vi "Scripting_ReplaceSubVI.vi"(8 "error in":errorcluster, 10 "NewVIToReplaceWith":path, 11 "CurrentSubVI":refnum<vi>) -> (0 "error out":errorcluster, 3 "ReplacedObject(SubVI)":refnum<vi>)   [LabVIEW 2016]
uses:
  <vilib>/Utility/miscctls.llb/LVPositionTypeDef.ctl
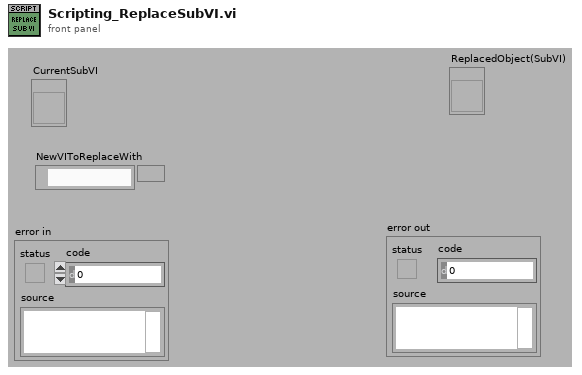
[diagram p1: front panel]
types:
  T1 = typedef "LVPositionTypeDef.ctl" = cluster{"Left":i32, "Top":i32}
  T2 = cluster{"ReplacedObject(SubVI)":refnum<vi>, "TerminalsOnCurrentSubVI":cluster{"Terminal":refnum<vi>, "Wire":refnum<vi>, "Position":T1, "IsSource":bool, "Data Type":variant, "WTerminals[]":refnum<vi>[]}[], "TerminalsOnNewSubVI":cluster{"Terminal":refnum<vi>, "Wire":refnum<vi>, "Position":T1, "IsSource":bool, "Data Type":variant, "WTerminals[]":refnum<vi>[]}[], "RepaireTerminals":cluster{"Org":cluster{"Terminal":refnum<vi>, "Wire":refnum<vi>, "Position":T1, "IsSource":bool, "Data Type":variant, "WTerminals[]":refnum<vi>[]}, "New":cluster{"Terminal":refnum<vi>, "Wire":refnum<vi>, "Position":T1, "IsSource":bool, "Data Type":variant, "WTerminals[]":refnum<vi>[]}}[]}
  T3 = cluster{"Terminal":refnum<vi>, "Wire":refnum<vi>, "Position":T1, "IsSource":bool, "Data Type":variant, "WTerminals[]":refnum<vi>[]}[]
  T4 = cluster{cluster{"Terminal":refnum<vi>, "Wire":refnum<vi>, "Position":T1, "IsSource":bool, "Data Type":variant, "WTerminals[]":refnum<vi>[]}, cluster{"Terminal":refnum<vi>, "Wire":refnum<vi>, "Position":T1, "IsSource":bool, "Data Type":variant, "WTerminals[]":refnum<vi>[]}}[]
  T5 = cluster{refnum<vi>, "Wire":refnum<vi>, "Position":T1, "IsSource":bool, "Data Type":variant, "Terms[]":refnum<vi>[]}
  T6 = cluster{"Terminal":refnum<vi>, "Wire":refnum<vi>, "Position":T1, "IsSource":bool, "Data Type":variant, "Terms[]":refnum<vi>[]}[]
  T7 = cluster{"Terminal":refnum<vi>, "Wire":refnum<vi>, "Position":T1, "IsSource":bool, "Data Type":variant, "WTerminals[]":refnum<vi>[]}
  T8 = cluster{cluster{"Terminal":refnum<vi>, "Wire":refnum<vi>, "Position":T1, "IsSource":bool, "Data Type":variant, "WTerminals[]":refnum<vi>[]}, cluster{"Terminal":refnum<vi>, "Wire":refnum<vi>, "Position":T1, "IsSource":bool, "Data Type":variant, "WTerminals[]":refnum<vi>[]}}
  T9 = cluster{"Org":cluster{"Terminal":refnum<vi>, "Wire":refnum<vi>, "Position":T1, "IsSource":bool, "Data Type":variant, "WTerminals[]":refnum<vi>[]}, "New":cluster{"Terminal":refnum<vi>, "Wire":refnum<vi>, "Position":T1, "IsSource":bool, "Data Type":variant, "WTerminals[]":refnum<vi>[]}}[]
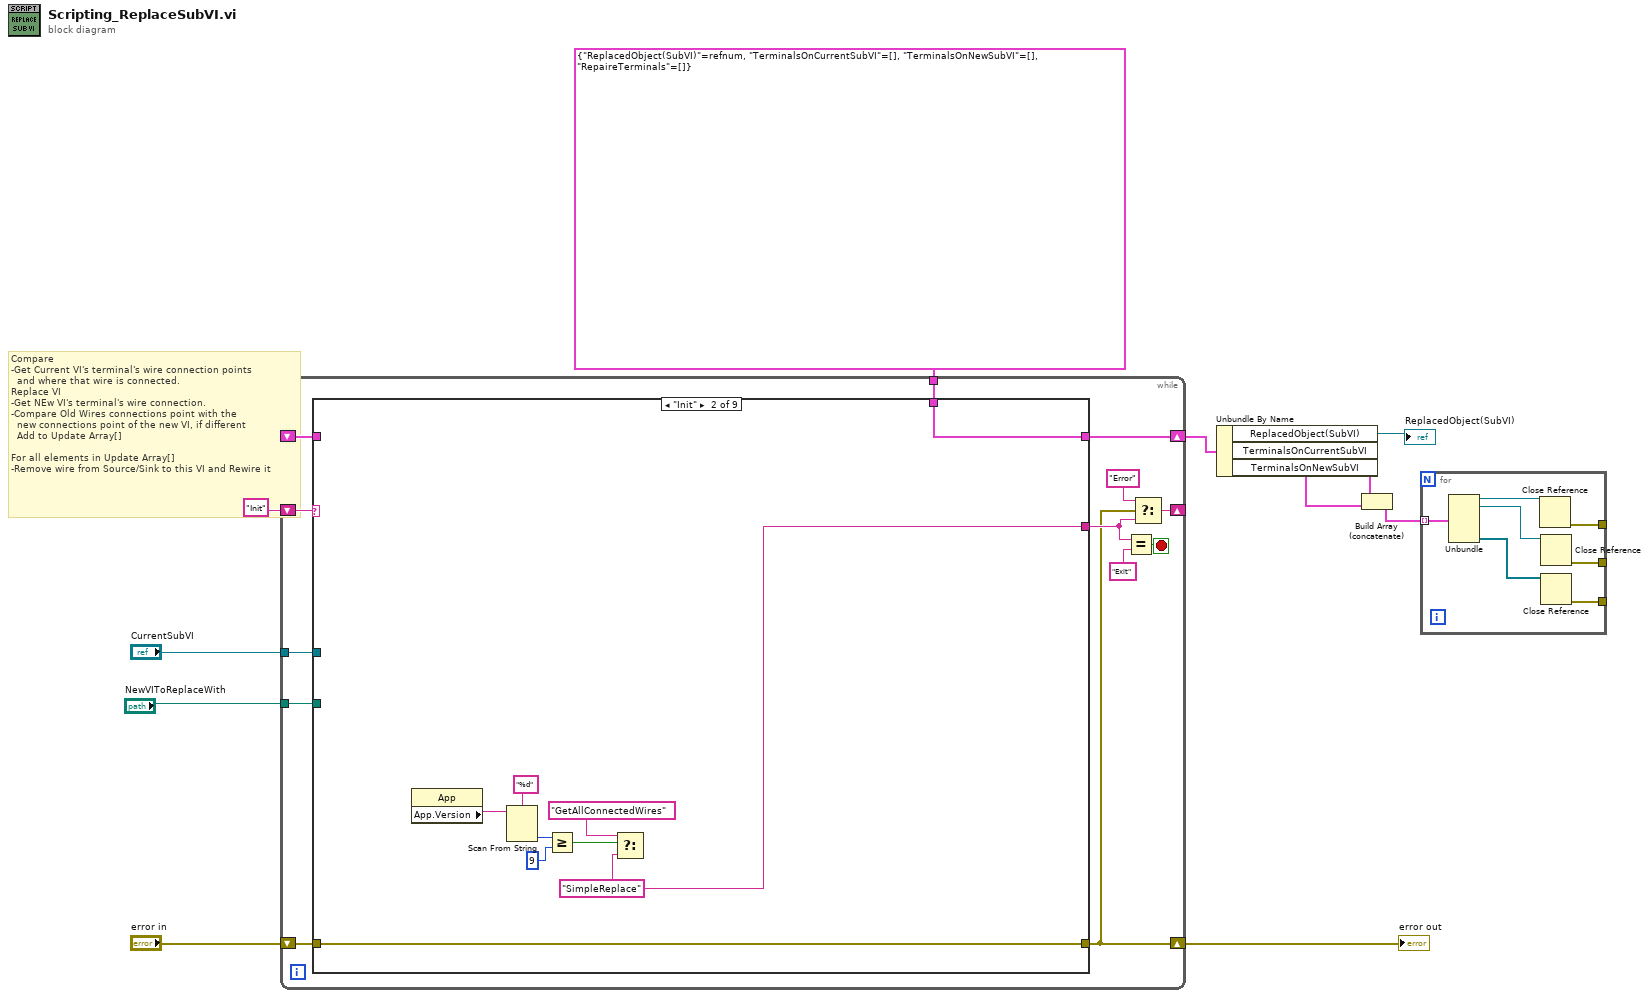
[diagram p0: block diagram]
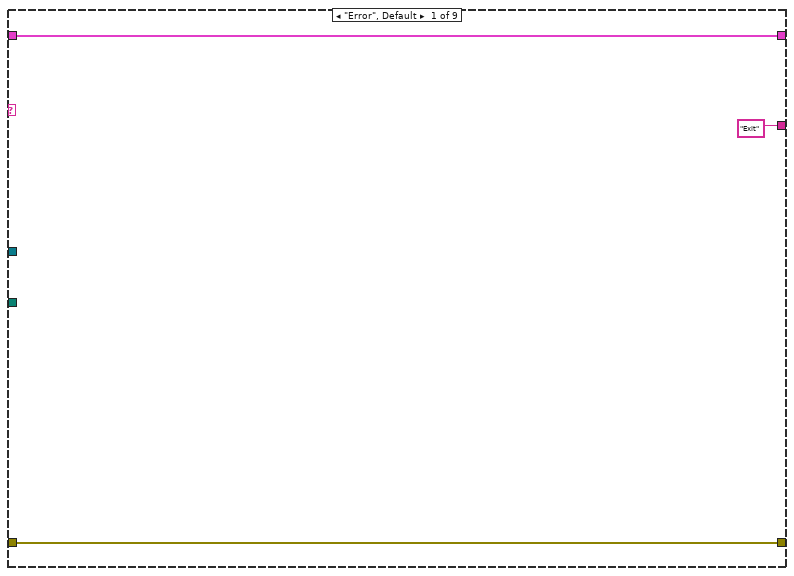
[diagram p2: hidden frame]
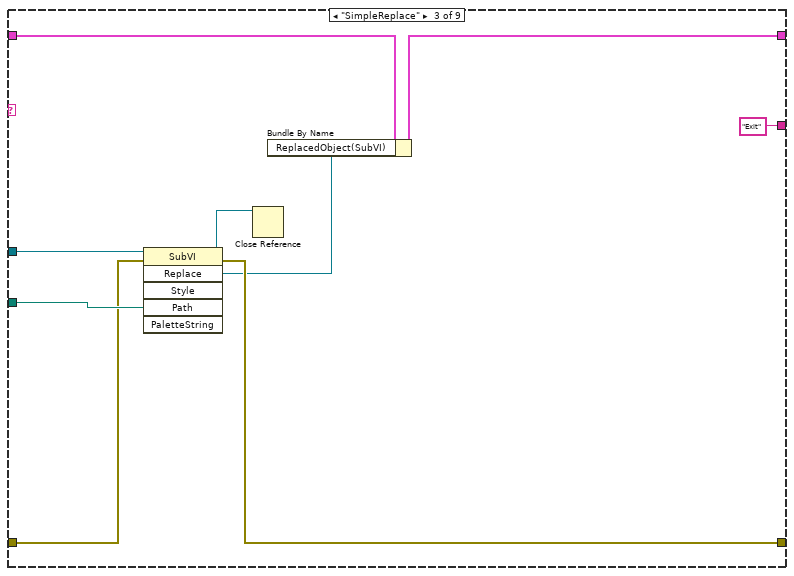
[diagram p3: hidden frame]
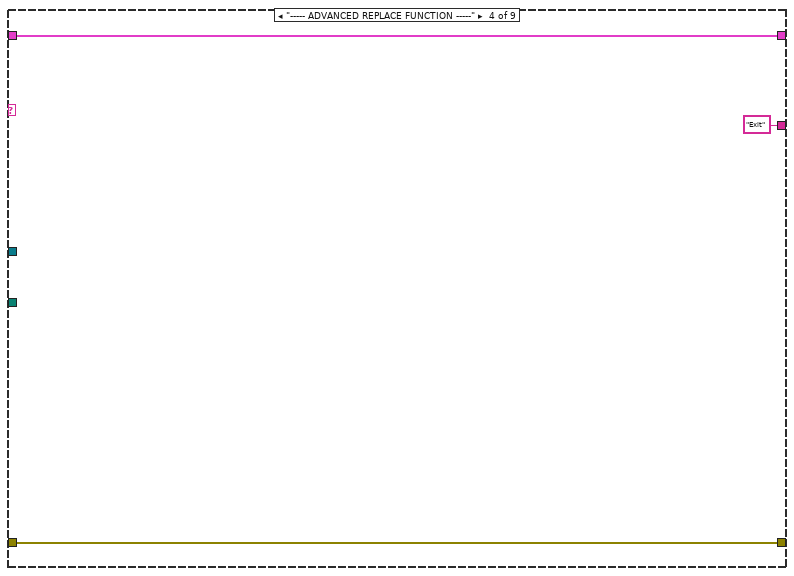
[diagram p4: hidden frame]
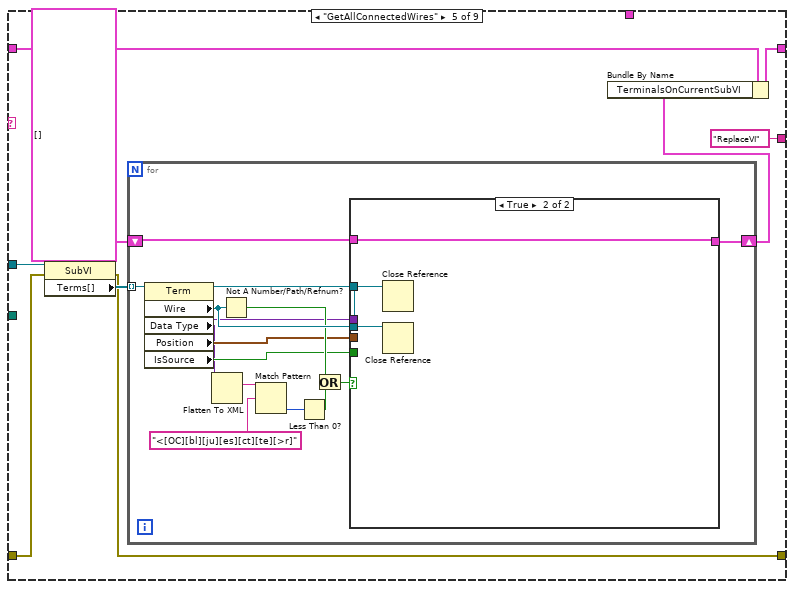
[diagram p5: hidden frame]
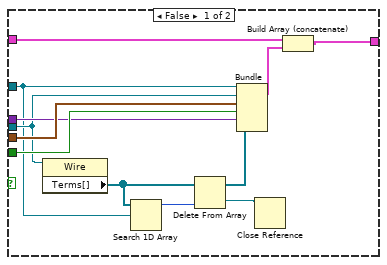
[diagram p6: hidden frame]
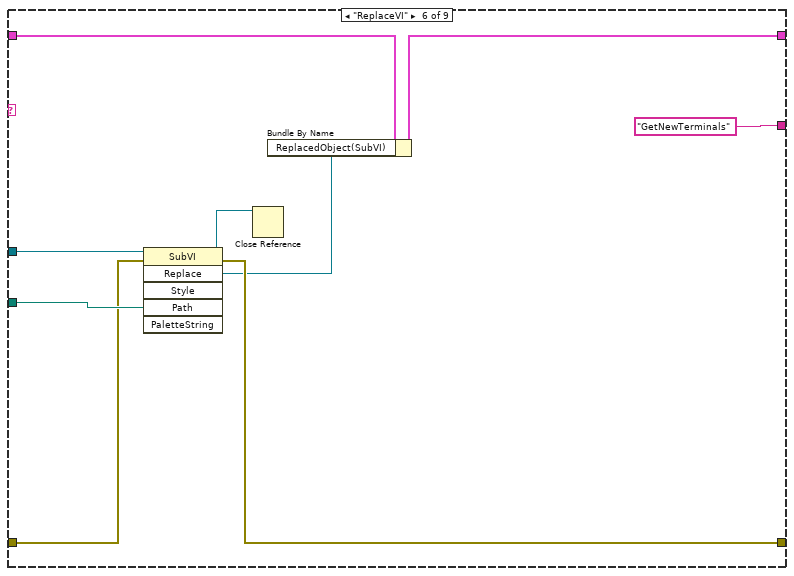
[diagram p7: hidden frame]
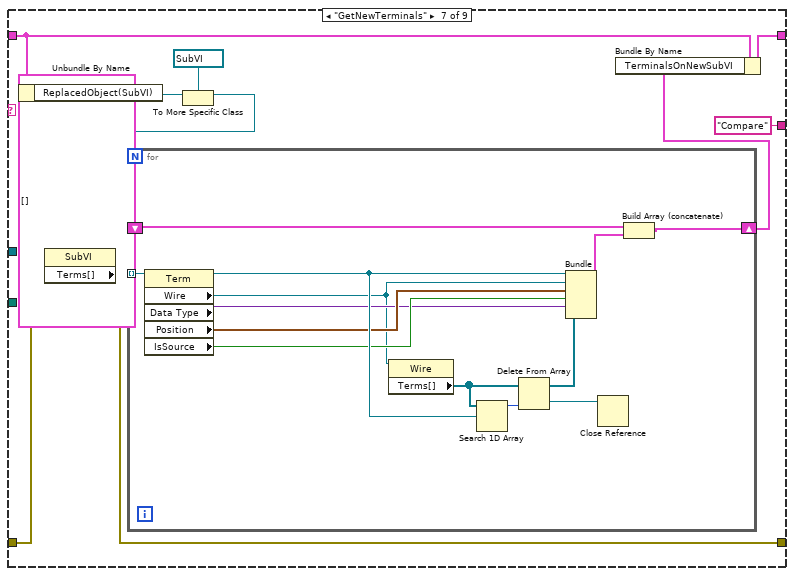
[diagram p8: hidden frame]
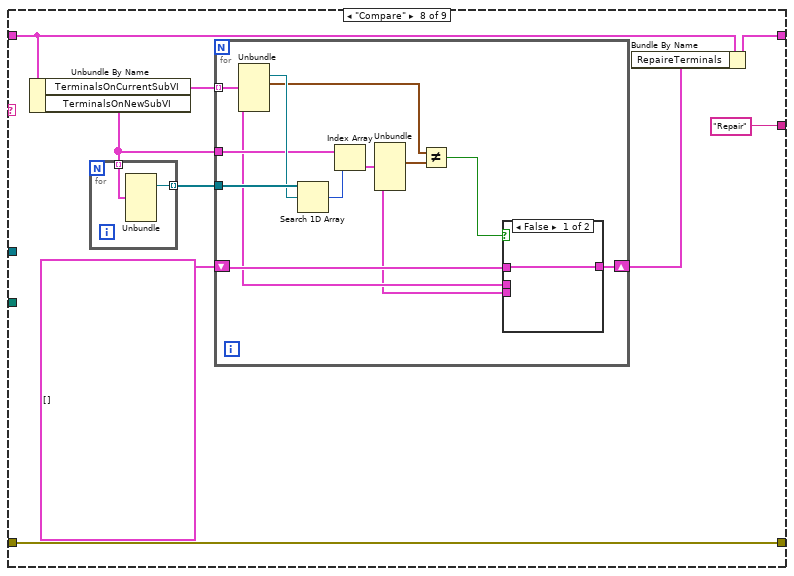
[diagram p9: hidden frame]
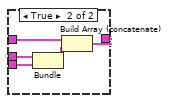
[diagram p10: hidden frame]
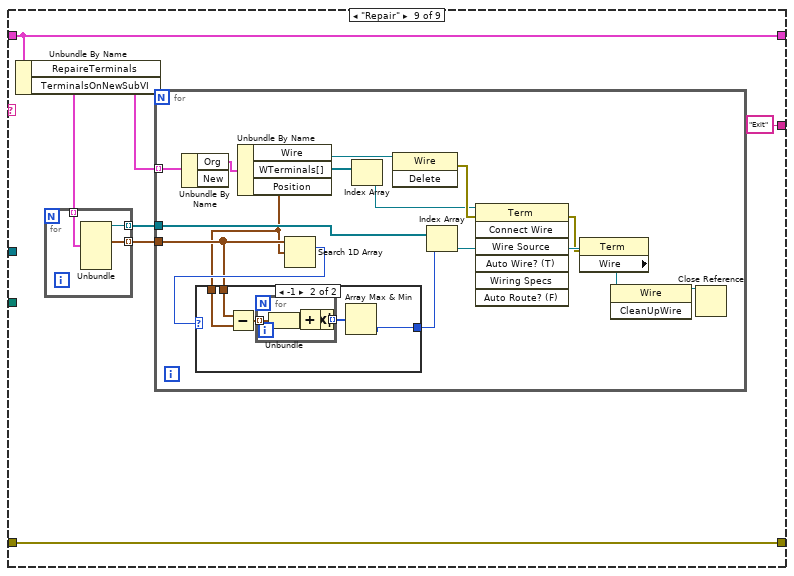
[diagram p11: hidden frame]
diagram:
  # "Compare\n-Get Current VI's terminal's wire connection points\n  and where that wire is connected.\nReplace VI\n-Get NEw VI's terminal's wire connection.\n-Compare Old Wires connections point with the\n  new connections point of the new VI, if different\n  Add to Update Array[]\n\nFor all elements in Update Array[]\n-Remove wire from Source/Sink to this VI and Rewire it"
  n1 = while {
    shift-right: [w17] -> w9
    shift-left: "error in" -> [w24]
    shift-right: [w22] -> _
    shift-left: "Init" -> [w23]
    shift-right: [w16] -> w8
    shift-left: _ -> [w15]
    tunnel: "CurrentSubVI" -> [w14]
    tunnel: "NewVIToReplaceWith" -> [w13]
    tunnel: T2 {"ReplacedObject(SubVI)"=refnum, "TerminalsOnCurrentSubVI"=[], "TerminalsOnNewSubVI"=[], "RepaireTerminals"=[]} -> [w12]
    stop <- w21 stop-if-true
    n2 = case shown="\"Init\"" w23 {
      tunnel: w24 -> [w27 w36 w41 w48 w56 w90 w105 w125 w152]
      tunnel: [w27 w36 w42 w48 w49 w91 w99 w125 w152] -> w17
      tunnel: ["Exit" w28 "Exit" "Exit" "ReplaceVI" ("f") "GetNewTerminals" "Compare" ("f") "Repair" "Exit"] -> w18
      tunnel: [w25 w29 w37 w47 w50 w86 w100 w119 w150] -> w16
      tunnel: w15 -> [w25 _ w39 w47 w52 w88 w98 w120 w150]
      tunnel: w14 -> [_ _ w44 _ w57 w93 _ _ _]
      tunnel: w13 -> [_ _ w43 _ _ w92 _ _ _]
      tunnel: w12 -> [_ w29 _ _ _ _ _ _ _]
      frame "Error", Default {
      }
      frame "Init" {
        w28 = "SimpleReplace" ("f")
        n3 = property class="App"() -> ("App.Version"=w35:string)  [unwired: 2 in, 2 out]
        n4 = Scan From String(format string="%d", input string=w35) -> (output 1=w33:i32)  [unwired: 3 in, 3 out]
        n5 = Greater Or Equal?(x=w33, y=9) -> (x >= y?=w31:bool)
        n6 = Select(t="GetAllConnectedWires", s=w31, f=w28) -> ()  [unwired: 1 out]
      }
      frame "SimpleReplace" {
        n7 = invoke class="SubVI" method="Replace"(reference=w44, error in=w41, "Path"=w43) -> (reference out=w45:refnum<vi>, error out=w42:errorcluster, "Replace"=w38:refnum<vi>)  [unwired: 3 in, 3 out]
        n8 = Close Reference(reference=w45) -> ()  [unwired: 1 in, 1 out]
        n9 = Bundle By Name(cluster=w39, "ReplacedObject(SubVI)"=w38) -> (w37:T2)
      }
      frame "----- ADVANCED REPLACE FUNCTION -----" {
      }
      frame "GetAllConnectedWires" {
        n10 = property class="SubVI"(reference=w57, error in=w56) -> (error out=w49:errorcluster, "Terms[]"=w55:refnum<vi>[])  [unwired: 1 out]
        n11 = for {
          tunnel: w55 -> [w71] mode=indexing
          shift-right: [w59] -> w51
          shift-left: T3 [] -> [w60]
          n12 = property class="Term"(reference=w71) -> (reference out=w63:refnum<vi>, "Wire"=w70:refnum<vi>, "Data Type"=w58:variant, "Position"=w62:T1, "IsSource"=w61:bool)  [unwired: 1 in, 1 out]
          n13 = Flatten To XML(anything=w58) -> (xml string=w69:string)
          n14 = Not A Number/Path/Refnum?(number/path/refnum=w70) -> (NaN/Path/Refnum?=w66:bool)
          n15 = Match Pattern(string=w69, regular expression="<[OC][bl][ju][es][ct][te][>r]") -> (offset past match=w67:i32)  [unwired: 1 in, 3 out]
          n16 = Less Than 0?(x=w67) -> (x < 0?=w65:bool)
          n17 = Or(x=w66, y=w65) -> (x .or. y?=w64:bool)
          n18 = case shown="True" w64 {
            tunnel: w70 -> [w77 _]
            tunnel: w63 -> [w76 w84]
            tunnel: w62 -> [w83 _]
            tunnel: w61 -> [w82 _]
            tunnel: w60 -> [w81 w85]
            tunnel: [w79 w85] -> w59
            tunnel: w58 -> [w78 _]
            frame False {
              n19 = property class="Wire"(reference=w77) -> ("Terms[]"=w75:refnum<vi>[])  [unwired: 1 in, 2 out]
              n20 = Search 1D Array(1D array=w75, element=w76) -> (index of element=w73:i32)  [unwired: 1 in]
              n21 = Delete From Array(array=w75, index=w73) -> (deleted portion=w72:refnum<vi>, array with subset deleted=w74:refnum<vi>[])  [unwired: 1 in]
              n22 = Bundle(w76, "Wire"=w77, "Position"=w83, "IsSource"=w82, "Data Type"=w78, "Terms[]"=w74) -> (w80:T5)  [unwired: 1 in]
              n23 = Close Reference(reference=w72) -> ()  [unwired: 1 in, 1 out]
              n24 = Build Array (concatenate)(w81, w80) -> (w79:T6)
            }
            frame True {
              n25 = Close Reference(reference=w84) -> ()  [unwired: 1 in, 1 out]
              n26 = Close Reference(reference=w84) -> ()  [unwired: 1 in, 1 out]
            }
          }
        }
        n27 = Bundle By Name(cluster=w52, "TerminalsOnCurrentSubVI"=w51) -> (w50:T2)
      }
      frame "ReplaceVI" {
        n28 = invoke class="SubVI" method="Replace"(reference=w93, error in=w90, "Path"=w92) -> (reference out=w94:refnum<vi>, error out=w91:errorcluster, "Replace"=w87:refnum<vi>)  [unwired: 3 in, 3 out]
        n29 = Close Reference(reference=w94) -> ()  [unwired: 1 in, 1 out]
        n30 = Bundle By Name(cluster=w88, "ReplacedObject(SubVI)"=w87) -> (w86:T2)
      }
      frame "GetNewTerminals" {
        n31 = Unbundle By Name(w98) -> ("ReplacedObject(SubVI)"=w97:refnum<vi>)
        n32 = To More Specific Class(target class=refnum<vi> refnum ("reference"), reference=w97) -> (specific class reference=w95:refnum<vi>)  [unwired: 1 in, 1 out]
        n33 = property class="SubVI"(reference=w95, error in=w105) -> (error out=w99:errorcluster, "Terms[]"=w104:refnum<vi>[])  [unwired: 1 out]
        n34 = for {
          tunnel: w104 -> [w118] mode=indexing
          shift-right: [w113] -> w101
          shift-left: T3 [] -> [w114]
          n35 = property class="Term"(reference=w118) -> (reference out=w117:refnum<vi>, "Wire"=w106:refnum<vi>, "Data Type"=w112:variant, "Position"=w116:T1, "IsSource"=w115:bool)  [unwired: 1 in, 1 out]
          n36 = property class="Wire"(reference=w106) -> ("Terms[]"=w110:refnum<vi>[])  [unwired: 1 in, 2 out]
          n37 = Search 1D Array(1D array=w110, element=w117) -> (index of element=w109:i32)  [unwired: 1 in]
          n38 = Delete From Array(array=w110, index=w109) -> (deleted portion=w107:refnum<vi>, array with subset deleted=w108:refnum<vi>[])  [unwired: 1 in]
          n39 = Bundle(w117, "Wire"=w106, "Position"=w116, "IsSource"=w115, "Data Type"=w112, "Terms[]"=w108) -> (w111:T5)  [unwired: 1 in]
          n40 = Close Reference(reference=w107) -> ()  [unwired: 1 in, 1 out]
          n41 = Build Array (concatenate)(w114, w111) -> (w113:T6)
        }
        n42 = Bundle By Name(cluster=w98, "TerminalsOnNewSubVI"=w101) -> (w100:T2)
      }
      frame "Compare" {
        n43 = Unbundle By Name(w120) -> ("TerminalsOnCurrentSubVI"=w127:T3, "TerminalsOnNewSubVI"=w123:T3)
        n44 = for {
          tunnel: w123 -> [w129] mode=indexing
          tunnel: [w128] -> w124 mode=indexing
          n45 = Unbundle(w129) -> ("Wire"=w128:refnum<vi>)  [unwired: 5 out]
        }
        n46 = for {
          tunnel: w127 -> [w133] mode=indexing
          tunnel: w123 -> [w138]
          tunnel: w124 -> [w140]
          shift-right: [w131] -> w121
          shift-left: T4 [] -> [w134]
          n47 = Unbundle(w133) -> ("Wire"=w139:refnum<vi>, "Position"=w135:T1)  [unwired: 4 out]
          n48 = Search 1D Array(1D array=w140, element=w139) -> (index of element=w137:i32)  [unwired: 1 in]
          n49 = Index Array(array=w138, index=w137) -> (element=w132:T7)
          n50 = Unbundle(w132) -> ("Position"=w136:T1)  [unwired: 5 out]
          n51 = Not Equal?(x=w135, y=w136) -> (x != y?=w130:bool)
          n52 = case shown="False" w130 {
            tunnel: w134 -> [w141 w146]
            tunnel: w133 -> [_ w145]
            tunnel: w132 -> [_ w144]
            tunnel: [w141 w142] -> w131
            frame False {
            }
            frame True {
              n53 = Bundle(w145, w144) -> (w143:T8)  [unwired: 1 in]
              n54 = Build Array (concatenate)(w146, w143) -> (w142:T4)
            }
          }
        }
        n55 = Bundle By Name(cluster=w120, "RepaireTerminals"=w121) -> (w119:T2)
      }
      frame "Repair" {
        n56 = Unbundle By Name(w150) -> ("RepaireTerminals"=w151:T9, "TerminalsOnNewSubVI"=w149:T3)
        n57 = for {
          tunnel: w149 -> [w156] mode=indexing
          tunnel: [w155] -> w148 mode=indexing
          tunnel: [w154] -> w147 mode=indexing
          n58 = Unbundle(w156) -> ("Terminal"=w154:refnum<vi>, "Position"=w155:T1)  [unwired: 4 out]
        }
        n59 = for {
          tunnel: w151 -> [w171] mode=indexing
          tunnel: w148 -> [w158]
          tunnel: w147 -> [w165]
          n60 = Unbundle By Name(w171) -> ("Org"=w170:T7)  [unwired: 1 out]
          n61 = Unbundle By Name(w170) -> ("Wire"=w168:refnum<vi>, "WTerminals[]"=w169:refnum<vi>[], "Position"=w157:T1)
          n62 = Search 1D Array(1D array=w158, element=w157) -> (index of element=w160:i32)  [unwired: 1 in]
          n63 = case shown="-1" w160 {
            selector: w160 -> [w172 _]
            tunnel: [w172 w173] -> w159
            tunnel: w158 -> [_ w177]
            tunnel: w157 -> [_ w176]
            frame 0, Default {
            }
            frame -1 {
              n64 = Subtract(x=w177, y=w176) -> (x-y=w175:T1[])
              n65 = for {
                tunnel: w175 -> [w182] mode=indexing
                tunnel: [w178] -> w174 mode=indexing
                n66 = Unbundle(w182) -> ("Left"=w181:i32, "Top"=w180:i32)
                n67 = Add(x=w181, y=w180) -> (x+y=w179:i32)
                n68 = Absolute Value(x=w179) -> (abs(x)=w178:i32)
              }
              n69 = Array Max & Min(array=w174) -> (min index (indices)=w173:i32)  [unwired: 3 out]
            }
          }
          n70 = Index Array(array=w169) -> (element=w166:refnum<vi>)  [unwired: 1 in]
          n71 = invoke class="Wire" method="Delete"(reference=w168) -> (error out=w167:errorcluster)  [unwired: 2 in, 2 out]
          n72 = Index Array(array=w165, index=w159) -> (element=w164:refnum<vi>)
          n73 = invoke class="Term" method="Connect Wire"(reference=w166, error in=w167, "Wire Source"=w164) -> (error out=w163:errorcluster)  [unwired: 4 in, 6 out]
          n74 = property class="Term"(reference=w164, error in=w163) -> ("Wire"=w162:refnum<vi>)  [unwired: 2 out]
          n75 = invoke class="Wire" method="CleanUpWire"(reference=w162) -> (reference out=w161:refnum<vi>)  [unwired: 2 in, 2 out]
          n76 = Close Reference(reference=w161) -> ()  [unwired: 1 in, 1 out]
        }
      }
    }
    n77 = Equal?(x=w18, y="Exit") -> (x = y?=w21:bool)
    n78 = Select(t="Error", s=w17, f=w18) -> (s? t:f=w22:string)
  }
  "error out" <- w9
  n79 = Unbundle By Name(w8) -> ("ReplacedObject(SubVI)"=→"ReplacedObject(SubVI)":refnum<vi>, "TerminalsOnCurrentSubVI"=w3:T3, "TerminalsOnNewSubVI"=w2:T3)
  n80 = Build Array (concatenate)(w3, w2) -> (w1:T3)
  n81 = for {
    tunnel: w1 -> [w189] mode=indexing
    tunnel: [w185] -> _
    tunnel: [w184] -> _
    tunnel: [w183] -> _
    n82 = Unbundle(w189) -> ("Terminal"=w188:refnum<vi>, "Wire"=w187:refnum<vi>, "WTerminals[]"=w186:refnum<vi>[])  [unwired: 3 out]
    n83 = Close Reference(reference=w188) -> (error out=w185:errorcluster)  [unwired: 1 in]
    n84 = Close Reference(reference=w187) -> (error out=w184:errorcluster)  [unwired: 1 in]
    n85 = Close Reference(reference=w186) -> (error out=w183:errorcluster)  [unwired: 1 in]
  }
